vi "SeqFileInit.vi"(8 "error in (no error)":errorcluster, 10 "RotateAngle":string, 11 "script path":string) -> (0 "error out":errorcluster, 4 "return":i32)   [LabVIEW 2019]
uses:
  ROI/Controls/ROI_List_Action.ctl
  [Global] ItemNames.vi
  [Global] RootPath.vi
  Caliper/Controls/Caliper_Entry_FGV_Action.ctl
  Coordinate/Control/CoordinateAction.ctl
  Controls/Parameter.ctl
  Caliper/Controls/CaliperResult.ctl
  Caliper/Controls/SelectionListEntryPointType.ctl
  Caliper/Controls/SelectionListEntry.ctl
  Caliper/Controls/CaliperType.ctl
  Caliper/Controls/CaliperDataEntry.ctl
  Controls/ParameterData.ctl
  Coordinate/Control/CoordinateAnalysisSetting.ctl
  Process/Controls/Process_Setting.ctl
  Coordinate/Control/CoordinatteEntry.ctl
  Analysis/Controls/Analysis_Setting.ctl
  Controls/Vision_DataEntry.ctl
  Controls/iVisionSEQ.ctl
  Coordinate/Control/CoordinateCaliperSetting.ctl
  Ctrl/VisionProcessName.ctl
  Analysis/Controls/V_Analysis_Type.ctl
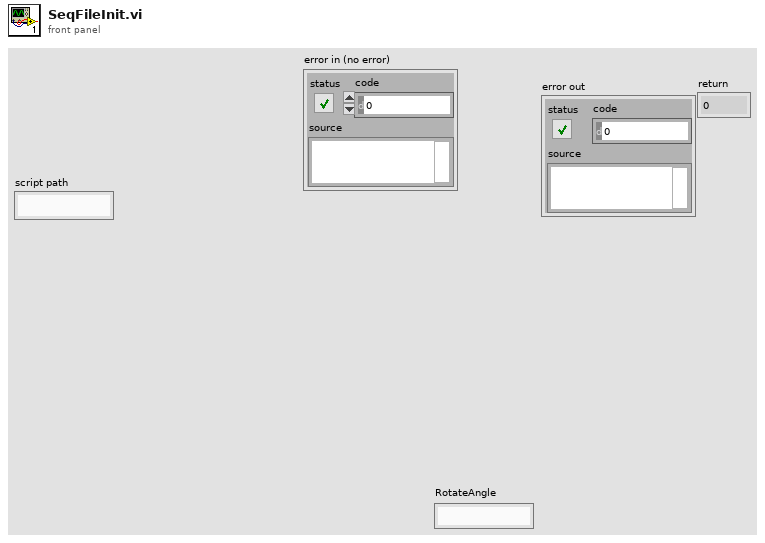
[diagram p1: front panel]
types:
  T1 = typedef "iVisionSEQ.ctl" = cluster{"iVision_Version":string, "iVisionSEQParam":variant}
  T2 = enum16{"open", "replace", "create", "open or create", "replace or create", "replace or create with confirmation"}
  T3 = typedef "Caliper_Entry_FGV_Action.ctl" = enum16{"Init", "Close", "Add", "Delete", "ReplaceAll", "ReadAll"}
  T4 = typedef "Parameter.ctl" = enum16{"Initialize", "Write", "Read", "WriteAll", "Save", "Load"}
  T5 = typedef "CoordinateAction.ctl" = enum16{"Initialize", "CoordEntryInput", "CoordEntryOutput", "CoordEntryTemp", "CoordEntryBackup", "CoordEntryReturn"}
  T6 = enum16{"Init", "Add", "Remove", "Read All", "Remove All"}
  T7 = typedef "ROI_List_Action.ctl" = enum16{"Init", "Add ROI", "Delete ROI", "Get All ROI", "Get Specific ROI", "Set Analysis Setting", "Set Process Setting", "Replace All Entries", "ROIEntryBackup", "ROIEntryBackupClear", "ROIEntryReturn"}
  T8 = typedef "ROI Descriptor" = cluster{"Global Rectangle":i32[], "Contours":cluster{"ID":enum32{"External", "Internal"}, "Type":u32, "Coordinates":i32[]}[]}
  T9 = cluster{"All ROI":cluster{"vROIName":string, "vROIContour":cluster{"Contour Type":u32, "ROI Type":u32, "Points":i32[]}, "ProcessSetting":cluster{"Process_Type":enum16{"None", "ExtractPlane", "BinaryMono", "Operators", "GrayMorphology", "Filters", "Lookup Table", "Particle Filter", "Mask"}, "Parameter":variant}[], "Analysis_Setting":cluster{"Analysis_Type":enum16{"None", "PatternMatch", "Edge Detection", "Barcode 1D", "Barcode 2D", "Clamp", "Clamp MAX", "Particle", "Histogram", "Straight Edge", "Circle", "Shape Dectect", "OCR"}, "RegionContour":cluster{"Contour Type":u32, "ROI Type":u32, "Points":i32[]}, "Parameter":variant}}[], "Output":cluster{"OutputList":u16[], "Criteria Condition":string[]}, string[][], "AllCaliperEntries":cluster{"CaliperType":u32, "Points":cluster{"Type":enum16{"AnalysisResult", "CaliperResult"}, "Index":i32}[], "Result":cluster{"PointInclude?":bool, "Num_Of_Pts":u8, "Position.X":dbl, "Position.Y":dbl, "Angle":dbl, "Distance":dbl, "Area":dbl, "Radius_MAX":dbl, "Radius2_min":dbl, "Dev_Residual":dbl, "P2.X":dbl, "P2.Y":dbl, "StepName":string, "Point ID":u8, "StepError?":bool, "ResultDiff?":bool}, "StepName":string}[], "CoordinatteEntry Output":cluster{"ProcessSetting":cluster{"Process_Type":enum16{"None", "ExtractPlane", "BinaryMono", "Operators", "GrayMorphology", "Filters", "Lookup Table", "Particle Filter", "Mask"}, "Parameter":variant}[], "Project Name":string, "AnalysisSetting":cluster{"Analysis_Type":enum16{"PatternMatch", "Straight Edge"}, "ROI ":T8, "Parameter":variant, "Step Result":variant, "OriginPointInfo":cluster{"Output Original":bool, "Origin Name":string, "Angle":dbl, "Mode":u16, "OriginPoint":cluster{"X":dbl, "Y":dbl}}, "AnalysisStepName":string}[], "Coord?":bool}, "ParameterData Out":cluster{"Rotate Angle":dbl, "Rotate?":bool, "Calibration File Path":string, "Cal?":bool}, "AllCaliperEntries":cluster{"CaliperType":u32, "Points":cluster{"Type":enum16{"AnalysisResult", "CaliperResult"}, "Index":i32}[], "Result":cluster{"PointInclude?":bool, "Num_Of_Pts":u8, "Position.X":dbl, "Position.Y":dbl, "Angle":dbl, "Distance":dbl, "Area":dbl, "Radius_MAX":dbl, "Radius2_min":dbl, "Dev_Residual":dbl, "P2.X":dbl, "P2.Y":dbl, "StepName":string, "Point ID":u8, "StepError?":bool, "ResultDiff?":bool}, "StepName":string}[]}
  T10 = typedef "Vision_DataEntry.ctl" = cluster{"vROIName":string, "vROIContour":cluster{"Contour Type":u32, "ROI Type":u32, "Points":i32[]}, "ProcessSetting":T11[], "Analysis_Setting":T13}
  T11 = typedef "Process_Setting.ctl" = cluster{"Enum_PreProcess":T12, "Parameter":string}
  T12 = typedef "VisionProcessName.ctl" = enum16{"*CamParameter*", "CamAttributes", "*Preprocess*", "CG_Brightness", "C_Plane Extraction", "C_Threshold", "G_Lookup Table", "G_Threshold", "B_Image Inversion"}
  T13 = typedef "Analysis_Setting.ctl" = cluster{"PreProcess":T14, "Parameter":string}
  T14 = typedef "V_Analysis_Type.ctl" = enum16{"None", "C_Color Pattern Matching", "G_PatternMatching", "G_ShapeDectect"}
  T15 = typedef "CaliperDataEntry.ctl" = cluster{"CaliperType":T16, "Points":T17[], "Result":T19, "StepName":string}
  T16 = typedef "CaliperType.ctl" = u32
  T17 = typedef "SelectionListEntry.ctl" = cluster{"Type":T18, "Index":i32}
  T18 = typedef "SelectionListEntryPointType.ctl" = enum16{"AnalysisResult", "CaliperResult"}
  T19 = typedef "CaliperResult.ctl" = cluster{"PointInclude?":bool, "Num_Of_Pts":u8, "Position.X":dbl, "Position.Y":dbl, "Angle":dbl, "Distance":dbl, "Area":dbl, "Radius_MAX":dbl, "Radius2_min":dbl, "Dev_Residual":dbl, "P2.X":dbl, "P2.Y":dbl, "StepName":string, "Point ID":u8, "StepError?":bool, "ResultDiff?":bool}
  T20 = typedef "CoordinatteEntry.ctl" = cluster{"ProcessSetting":T11[], "Project Name":string, "AnalysisSetting":T21[], "Coord?":bool, "OriginPointInfo":cluster{"Output Original":bool, "Origin Name":string, "Angle":dbl, "Mode":u16, "OriginPoint":cluster{"X":dbl, "Y":dbl}}, "CaliperSetting":T22[], "CoordIndex":i32[]}
  T21 = typedef "CoordinateAnalysisSetting.ctl" = cluster{"Analysis_Type":enum16{"PatternMatch", "Straight Edge"}, "ROI ":T8, "Parameter":variant, "Step Result":variant, "AnalysisStepName":string, "CoordinateUse":bool}
  T22 = typedef "CoordinateCaliperSetting.ctl" = cluster{"Result":variant, "CoordinateUse":bool, "CaliperEntry":T15}
  T23 = typedef "ParameterData.ctl" = cluster{"Rotate Angle":dbl, "Rotate?":bool, "Calibration File Path":string, "Cal?":bool}
  T24 = cluster{"All ROI":T10[], "Output":cluster{"OutputList":u16[], "Criteria Condition":string[]}, string[][], "AllCaliperEntries":T15[], "CoordinatteEntry Output":T20, "ParameterData Out":T23, "AllCaliperEntries":T15[]}
  T25 = cluster{"OutputList":u16[], "Criteria Condition":string[]}
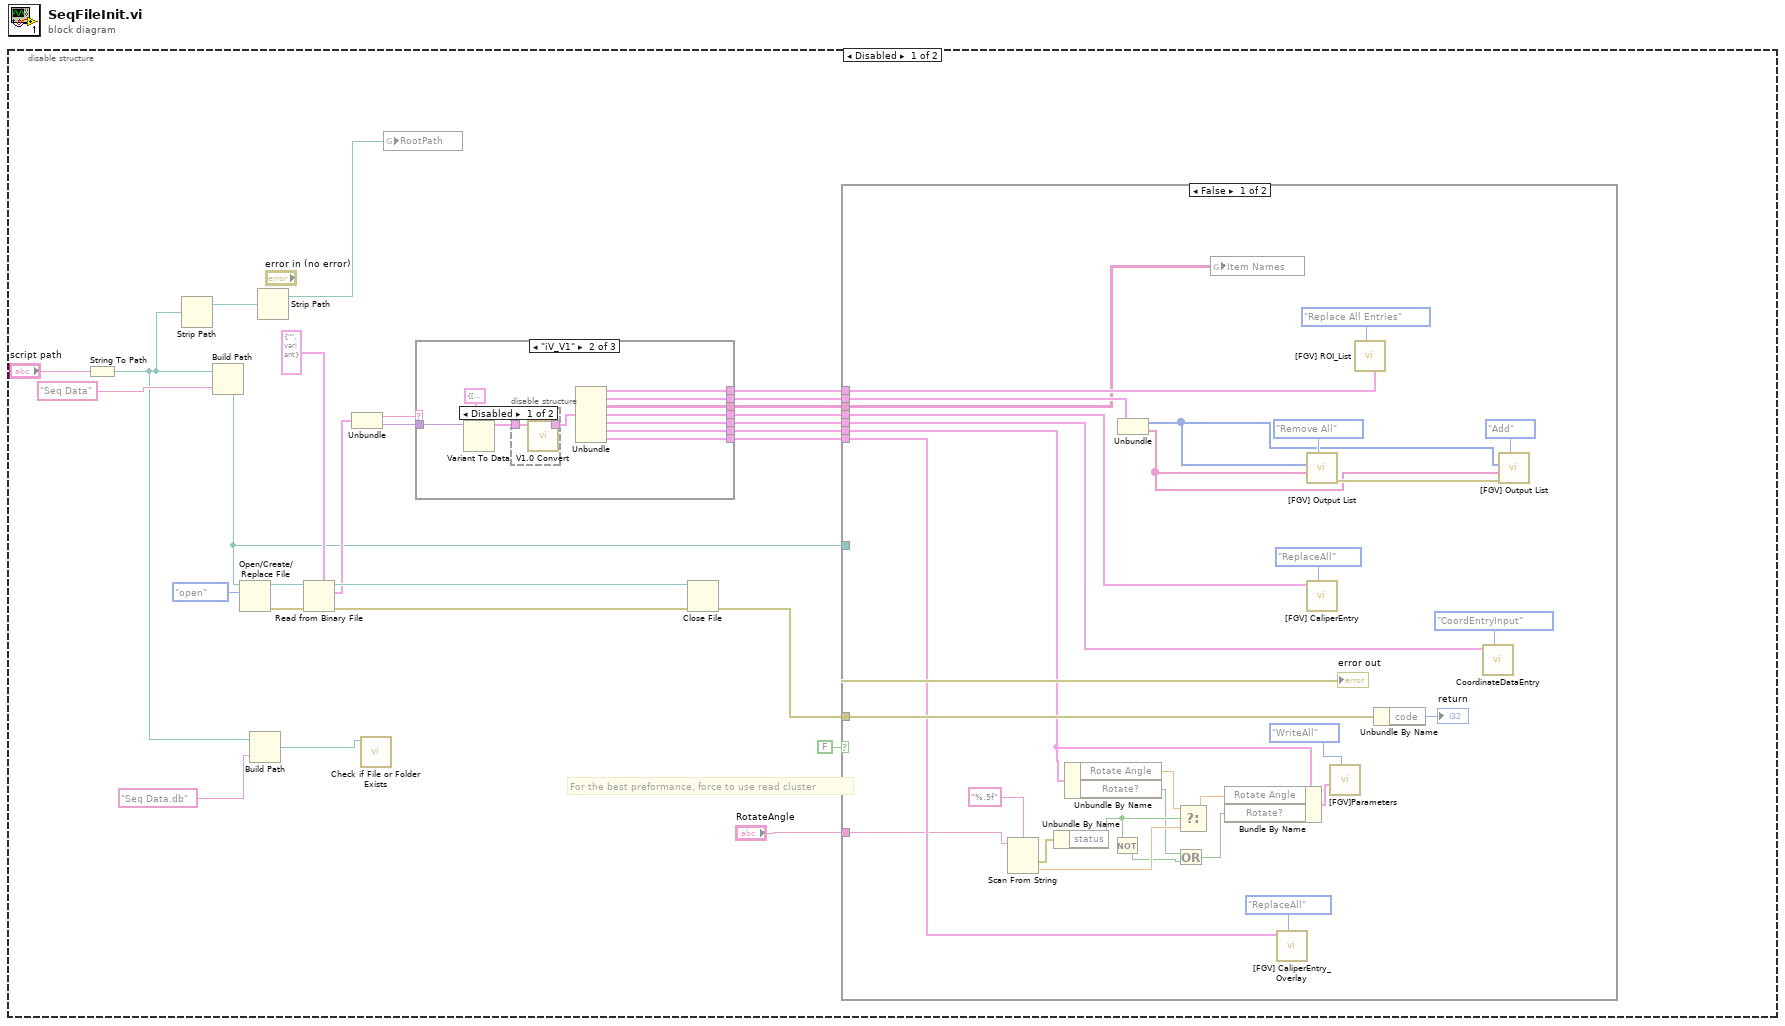
[diagram p0: block diagram]
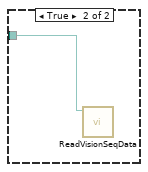
[diagram p2: hidden frame]
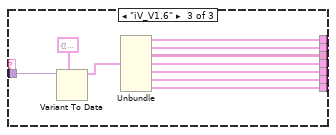
[diagram p5: hidden frame]
diagram:
  n1 = disable-structure shown="Disabled" {
    frame Disabled {
      # "For the best preformance, force to use read cluster"
      n2 = String To Path(string="script path") -> (path=w6:path)
      n3 = Strip Path(path=w6) -> (stripped path=w18:path)  [unwired: 1 out]
      n4 = Build Path(base path=w6, name or relative path="Seq Data") -> (appended path=w3:path)
      n5 = Open/Create/Replace File(file path (use dialog)=w3, operation (0:open)=T2."open") -> (refnum out=w24:refnum<file>, error out=w27:errorcluster)  [unwired: 4 in, 1 out]
      n6 = Build Path(base path=w6, name or relative path="Seq Data.db") -> (appended path=w4:path)
      n7 = Strip Path(path=w18) -> (stripped path=w17:path)  [unwired: 1 out]
      n8 = Read from Binary File(5:T1 {"iVision_Version"="", "iVisionSEQParam"=variant} ("iVisionSEQ"), 8:w27, 11:w24) -> (0:w26:errorcluster, 2:w10:T1, 3:w23:refnum<file>)  [unwired: 3 in, 1 out]
      n9 = Unbundle(w10) -> ("iVision_Version"=w9:string, "iVisionSEQParam"=w8:variant)
      n10 = call <vilib>:"Check if File or Folder Exists.vi"("path"=w4) -> ()  [unwired: 8 in, 3 out]
      n11 = global write "[Global] RootPath.vi" "RootPath"(w17) -> ()
      n12 = case shown="\"iV_V1\"" w9 {
        tunnel: [_ w65 w81] -> w20
        tunnel: [_ w62 w80] -> w16
        tunnel: [_ w64 w79] -> w15
        tunnel: [_ w61 w78] -> w14
        tunnel: [_ w60 w77] -> w7
        tunnel: [_ w59 w76] -> w13
        tunnel: [_ w63 w75] -> w12
        tunnel: w8 -> [_ w67 w74]
        frame "False", Default {
        }
        frame "iV_V1" {
          n13 = Variant To Data(type=T9 {"All ROI"=[], "Output"={"OutputList"=[], "Criteria Condition"=[]}, [], "AllCaliperEntries"=[], "CoordinatteEntry Output"={"ProcessSetting"=[], "Project Name"="", "AnalysisSetting"=[], "Coord?"=FALSE}, "ParameterData Out"={"Rotate Angle"=0.0, "Rotate?"=FALSE, "Calibration File Path"="", "Cal?"=FALSE}, "AllCaliperEntries"=[]} ("Old"), Variant=w67) -> (data=w69:T9)  [unwired: 1 in, 1 out]
          n14 = disable-structure shown="Disabled" {
            disable-tunnel: w69 -> [w71 _]
            disable-tunnel: [w70 _] -> w66
            frame Disabled {
              n15 = call "V1.0 Convert.vi"("Old"=w71) -> ("NewOut"=w70:T24)  [unwired: 10 in]
            }
            frame Enabled {
            }
          }
          n16 = Unbundle(w66) -> ("All ROI"=w65:T10[], "Output"=w64:T25, w63:string[][], "AllCaliperEntries"=w62:T15[], "CoordinatteEntry Output"=w61:T20, "ParameterData Out"=w60:T23, "AllCaliperEntries"=w59:T15[])
        }
        frame "iV_V1.6" {
          n17 = Variant To Data(type=T24 {"All ROI"=[], "Output"={"OutputList"=[], "Criteria Condition"=[]}, [], "AllCaliperEntries"=[], "CoordinatteEntry Output"={"ProcessSetting"=[], "Project Name"="", "AnalysisSetting"=[], "Coord?"=FALSE, "OriginPointInfo"={"Output Original"=FALSE, "Origin Name"="", "Angle"=0.0, "Mode"=0, "OriginPoint"={"X"=0.0, "Y"=0.0}}, "CaliperSetting"=[], "CoordIndex"=[]}, "ParameterData Out"={"Rotate Angle"=0.0, "Rotate?"=FALSE, "Calibration File Path"="", "Cal?"=FALSE}, "AllCaliperEntries"=[]} ("output cluster"), Variant=w74) -> (data=w72:T24)  [unwired: 1 in, 1 out]
          n18 = Unbundle(w72) -> ("All ROI"=w81:T10[], "Output"=w79:T25, w75:string[][], "AllCaliperEntries"=w80:T15[], "CoordinatteEntry Output"=w78:T20, "ParameterData Out"=w77:T23, "AllCaliperEntries"=w76:T15[])
        }
      }
      n19 = Close File(refnum=w23, error in=w26) -> (error out=w19:errorcluster)  [unwired: 1 out]
      n20 = case shown="False" FALSE {
        tunnel: w20 -> [w54 _]
        tunnel: w19 -> [w51 _]
        tunnel: w16 -> [w49 _]
        tunnel: w15 -> [w48 _]
        tunnel: w14 -> [w47 _]
        tunnel: w13 -> [w44 _]
        tunnel: w12 -> [w41 _]
        tunnel: w7 -> [w39 _]
        tunnel: w3 -> [_ w58]
        tunnel: "RotateAngle" -> [w28 _]
        frame False {
          n21 = Scan From String(format string="%.5f", input string=w28) -> (error out=w35:errorcluster, output 1=w33:dbl)  [unwired: 3 in, 2 out]
          n22 = Unbundle By Name(w35) -> ("status"=w32:bool)
          n23 = Unbundle By Name(w39) -> ("Rotate Angle"=w40:dbl, "Rotate?"=w31:bool)
          n24 = Not(x=w32) -> (.not. x?=w29:bool)
          n25 = Unbundle(w48) -> ("OutputList"=w43:u16[], "Criteria Condition"=w42:string[])
          n26 = Or(x=w31, y=w29) -> (x .or. y?=w30:bool)
          n27 = Select(t=w40, s=w32, f=w33) -> (s? t:f=w37:dbl)
          n28 = global write "[Global] ItemNames.vi" "Item Names"(w41) -> ()
          n29 = Bundle By Name(cluster=w39, "Rotate Angle"=w37, "Rotate?"=w30) -> (w36:T23)
          n30 = call "[FGV] CaliperEntry_Overlay.vi"("Action"=Caliper_Entry_FGV_Action."ReplaceAll", "CaliperEntriesIn"=w44) -> ()  [unwired: 8 in, 2 out]
          n31 = call "[FGV] Output List.vi"("Action"=T6."Remove All", "Criteria"=w42, "Indexes In"=w43) -> ("error out"=w53:errorcluster)  [unwired: 7 in, 1 out]
          n32 = call "[FGV] CaliperEntry.vi"("Action"=Caliper_Entry_FGV_Action."ReplaceAll", "CaliperEntriesIn"=w49) -> ()  [unwired: 8 in, 2 out]
          n33 = call "[FGV]Parameters.vi"("Parameter"=Parameter."WriteAll", "ParameterData In"=w36) -> ()  [unwired: 8 in, 2 out]
          n34 = call "[FGV] ROI_List.vi"("ROIEntriesIn"=w54, "Action"=ROI_List_Action."Replace All Entries") -> ()  [unwired: 7 in, 3 out]
          n35 = Unbundle By Name(w51) -> ("code"=→"return":i32)
          n36 = call "CoordinateDataEntry.vi"("CoordinateAction"=CoordinateAction."CoordEntryInput", "OneCoordStep Input"=w47) -> ()  [unwired: 8 in, 2 out]
          n37 = call "[FGV] Output List.vi"("Action"=T6."Add", "error in (no error)"=w53, "Criteria"=w42, "Indexes In"=w43) -> ()  [unwired: 6 in, 2 out]
          "error out" <- w51
        }
        frame True {
          n38 = call "ReadVisionSeqData.vi"("SeqDataPath"=w58) -> ()  [unwired: 9 in, 2 out]
        }
      }
    }
    frame Enabled {
    }
  }
